vi "Read Results.vi"(8 "error in (no error)":errorcluster, 11 "Hardware in":refnum<class "Hardware.lvclass">) -> (0 "error out":errorcluster, 2 "Results":refnum<class "Hardware Result.lvclass">[](array[class]), 3 "Hardware out":refnum<class "Hardware.lvclass">)   [LabVIEW 2018, in "Hardware.lvclass"]
uses:
  Hardware.lvclass
  Hardware Result Class/Hardware Result.lvclass
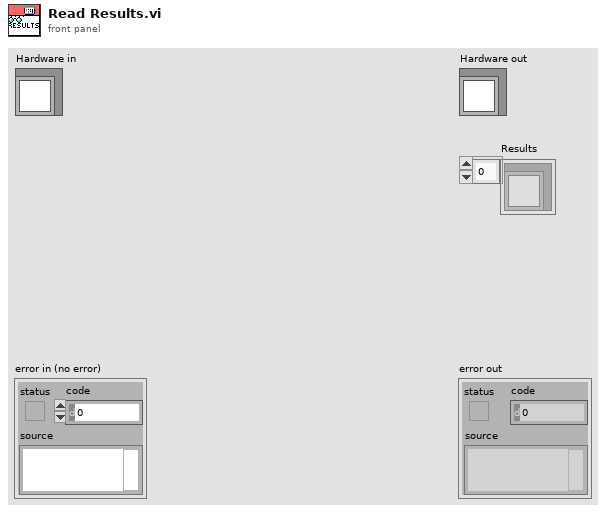
[diagram p1: front panel]
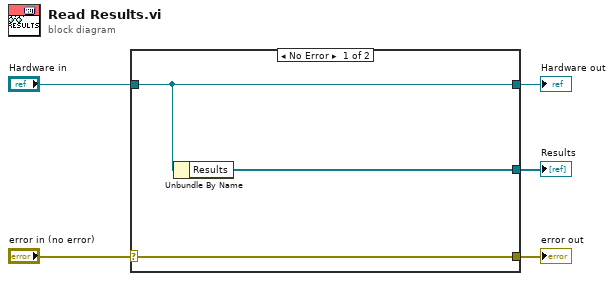
[diagram p0: block diagram]
diagram:
  n1 = case shown="No Error" "error in (no error)" {
    selector: "error in (no error)" -> [w8 w9]
    tunnel: [w8 w9] -> w4
    tunnel: [w7 w10] -> w2
    tunnel: "Hardware in" -> [w7 w10]
    tunnel: [w6 _] -> w1
    frame No Error {
      n2 = Unbundle By Name(w7) -> ("Results"=w6:refnum<class "Hardware Result.lvclass">[])
    }
    frame Error {
    }
  }
  "error out" <- w4
  "Hardware out" <- w2
  "Results" <- w1
